vi "Execute.vi"(6 "WhereIGetMyInformationDescription":string, 8 "error in (no error)":errorcluster caption="Fehler (Eingang, kein Fehler)", 9 "WhereIGetMyInformation":string, 10 "WhoIAm":string, 11 "LoadConfigurationDataBase Eingang":refnum<class "LoadConfigurationDataBase.lvclass"> caption="DNL_LabVIEW Object in") -> (0 "error out":errorcluster caption="Fehler (Ausgang)", 2 "LvDictionary.lvlib:DictionaryString.lvclass":refnum<class "DictionaryString.lvclass">, 3 "LoadConfigurationDataBase Ausgang":refnum<class "LoadConfigurationDataBase.lvclass"> caption="DNL_LabVIEW Object out")   [LabVIEW 2013, in "LoadConfigurationDataBase.lvclass"]
uses:
  LoadConfigurationDataBase.lvclass
  LvDictionary/DictionaryStringClass/DictionaryString.lvclass
  System.Data
panel:
  out "Array":string[][](array[string])
  out "Count 2":i32
  out "Count":i32
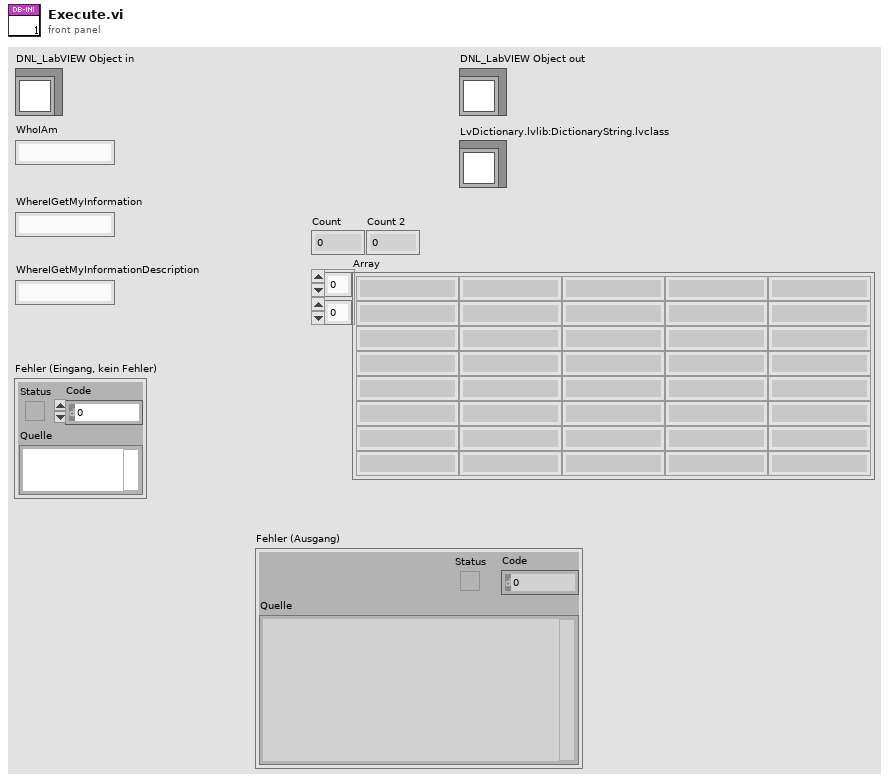
[diagram p1: front panel]
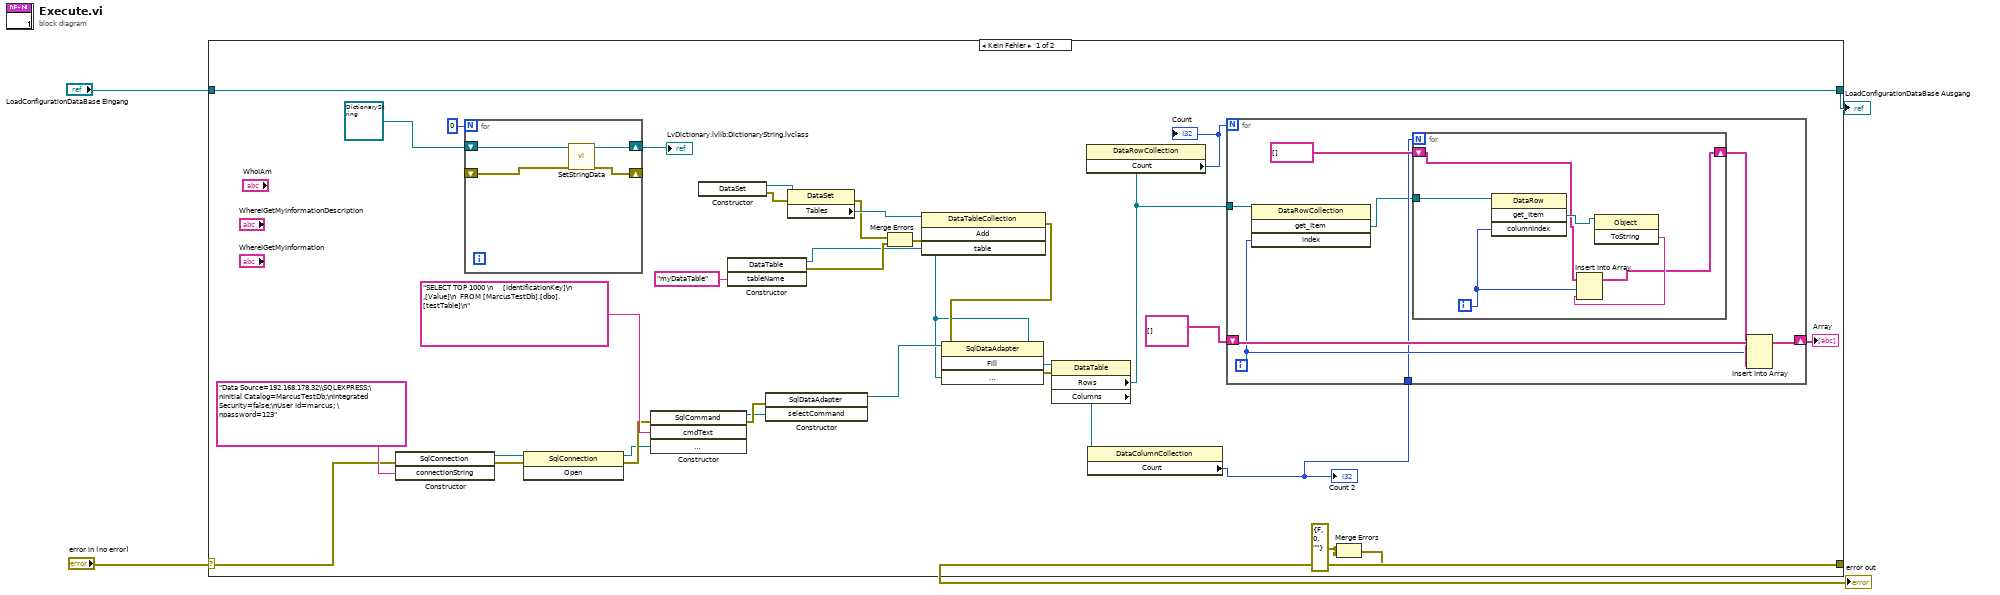
[diagram p0: block diagram]
diagram:
  n1 = case shown="Kein Fehler" "error in (no error)" {
    selector: "error in (no error)" -> [w28 w56]
    tunnel: [w21 w56] -> w3
    tunnel: [w36 w55] -> w1
    tunnel: "LoadConfigurationDataBase Eingang" -> [w36 w55]
    frame No Error {
      w10 = errorcluster {"status"=FALSE, "code"=0, "source"=""} ("Fehler (Eingang)")
      n2 = constructor class="SqlConnection"(error in=w28, "connectionString"="Data Source=192.168.178.32\\SQLEXPRESS;\nInitial Catalog=MarcusTestDb;\nIntegrated Security=false;\nUser Id=marcus; \npassword=123") -> (reference out=w32:refnum<k24>, error out=w31:errorcluster)  [unwired: 2 in, 2 out]
      n3 = for {
        N: 0 -> [_]
        shift-right: [w52] -> w34
        shift-left: refnum<class "DictionaryString.lvclass"> refnum ("LvDictionary.lvlib:DictionaryString.lvclass") -> [w54]
        shift-right: [w51] -> _
        shift-left: _ -> [w53]
        n4 = call-dynamic "SetStringData.vi"("error in (no error)"=w53, "DictionaryString Eingang"=w54) -> ("error out"=w51:errorcluster, "DictionaryString Ausgang"=w52:refnum<class "DictionaryString.lvclass">)  [unwired: 8 in]
      }
      "LvDictionary.lvlib:DictionaryString.lvclass" <- w34
      n5 = invoke on="Methodenknoten" class="SqlConnection" method="Open"(reference=w32, error in=w31) -> (reference out=w24:refnum<k24>, error out=w29:errorcluster)  [unwired: 1 in, 1 out]
      n6 = constructor class="SqlCommand"(error in=w29, "cmdText"="SELECT TOP 1000 \n     [IdentificationKey]\n      ,[Value]\n  FROM [MarcusTestDb].[dbo].[testTable]\n", "connection"=w24) -> (reference out=w25:refnum<k24>, error out=w27:errorcluster)  [unwired: 2 in, 3 out]
      n7 = constructor class="DataSet"() -> (reference out=w19:refnum<k24>, error out=w18:errorcluster)  [unwired: 3 in, 1 out]
      n8 = constructor class="DataTable"("tableName"="myDataTable") -> (reference out=w12:refnum<k24>, error out=w14:errorcluster)  [unwired: 3 in, 2 out]
      n9 = constructor class="SqlDataAdapter"(error in=w27, "selectCommand"=w25) -> (reference out=w23:refnum<k24>)  [unwired: 2 in, 3 out]
      n10 = property class="DataSet"(reference=w19, error in=w18) -> (error out=w16:errorcluster, "Tables"=w17:refnum<k24>)  [unwired: 1 out]
      n11 = Merge Errors(w16, w14) -> (w15:errorcluster)
      n12 = invoke class="DataTableCollection" method="Add"(reference=w17, error in=w15, "table"=w12) -> (error out=w13:errorcluster)  [unwired: 1 in, 3 out]
      n13 = invoke class="SqlDataAdapter" method="Fill"(reference=w23, error in=w13, "dataTable"=w12) -> (error out=w22:errorcluster)  [unwired: 1 in, 3 out]
      n14 = property class="DataTable"(reference=w12, error in=w22) -> ("Rows"=w8:refnum<k24>, "Columns"=w11:refnum<k24>)  [unwired: 2 out]
      n15 = property class="DataRowCollection"(reference=w8) -> ("Count"=w9:i32)  [unwired: 1 in, 2 out]
      "Count" <- w9
      n16 = property class="DataColumnCollection"(reference=w11) -> ("Count"=w6:i32)  [unwired: 1 in, 2 out]
      "Count 2" <- w6
      n17 = for {
        N: w9 -> [_]
        tunnel: w8 -> [w44]
        shift-right: [w43] -> w5
        shift-left: string[][] [] -> [w42]
        tunnel: w6 -> [w38]
        i -> [w39]
        n18 = invoke class="DataRowCollection" method="get_Item"(reference=w44, "index"=w39) -> ("get_Item"=w37:refnum<k24>)  [unwired: 2 in, 3 out]
        n19 = for {
          N: w38 -> [_]
          shift-right: [w45] -> w40
          shift-left: string[] [] -> [w46]
          tunnel: w37 -> [w50]
          i -> [w49]
          n20 = invoke class="DataRow" method="get_Item"(reference=w50, "columnIndex"=w49) -> ("get_Item"=w48:refnum<k24>)  [unwired: 2 in, 3 out]
          n21 = invoke class="Object" method="ToString"(reference=w48) -> ("ToString"=w47:string)  [unwired: 2 in, 2 out]
          n22 = Insert Into Array(array=w46, index=w49, new element=w47) -> (w45:string[])
        }
        n23 = Insert Into Array(array=w42, index (row)=w39, new element=w40) -> (w43:string[][])  [unwired: 1 in]
      }
      "Array" <- w5
      n24 = Merge Errors(w10, w10) -> (w21:errorcluster)
    }
    frame Error {
    }
  }
  "error out" <- w3
  "LoadConfigurationDataBase Ausgang" <- w1
